vi "Dispose.vi"(8 "error in":errorcluster, 11 "NYStyleCheesePizza":refnum<class "NYStyleCheesePizza.lvclass">) -> (0 "error out":errorcluster)   [LabVIEW 2020, in "FactoryMethod.lvlib" / "PizzaFactoryMethod.lvlib" / "NYStyleCheesePizza.lvclass"]
uses:
  NYStyleCheesePizza.lvclass
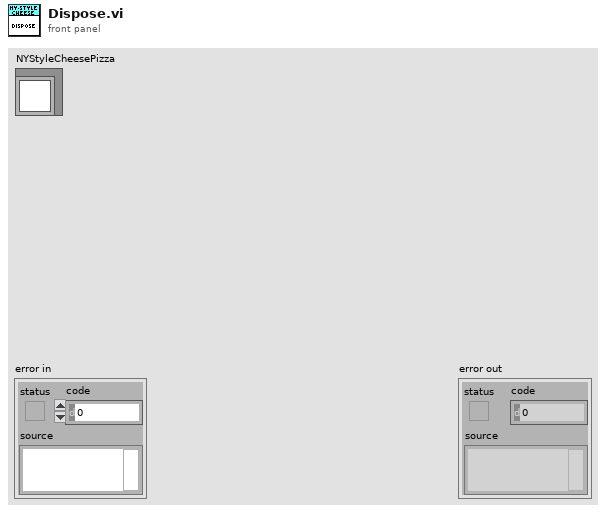
[diagram p1: front panel]
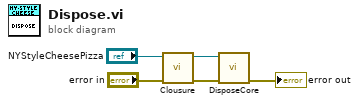
[diagram p0: block diagram]
diagram:
  n1 = call-dynamic "Clousure.vi"("error in"="error in", "NYStyleCheesePizza"="NYStyleCheesePizza") -> ("error out"=w3:errorcluster, "NYStyleCheesePizza"=w4:refnum<class "NYStyleCheesePizza.lvclass">)  [unwired: 8 in]
  n2 = call-dynamic "DisposeCore.vi"("error in (no error)"=w3, "NYStyleCheesePizza"=w4) -> ("error out"=→"error out":errorcluster)  [unwired: 8 in, 1 out]
